vi "Initialize.vi"(8 "error in (no error)":errorcluster, 9 "id query (False)":bool caption="id query (True)", 10 "reset device (False)":bool caption="reset device (True)", 11 "Simulation in":refnum<class "Simulation.lvclass">) -> (0 "error out":errorcluster, 3 "Simulation out":refnum<class "Simulation.lvclass">)   [LabVIEW 2018, in "DigitizerPlugins.lvlib" / "Simulation.lvclass"]
uses:
  Simulation.lvclass
  Y:/Projects/PMUCal/Modules/Digitizer/DigitizerPlugins/DigitizerBaseClass/DigitizerBase.lvclass
  FGen/MemberClasses/PmuTestFunctions/PmuTestConfig.ctl
  FGen/MemberClasses/ArbitraryFunction/TypeDefs/ArbCfg.ctl
  FGen/MemberClasses/ArbitraryFunction/TypeDefs/Arbitrary.ctl
  Simulation.lvclass/Simulation.ctl
  DigitizerBaseClass/DigitizerBase.lvclass/DigitizerBase.ctl
  Accessors/Read Function.vi
  DigitizerBaseClass/Accessors/Read Acquisition.vi
  Accessors/Write Function.vi
  FGen/MemberClasses/FunctionBaseClass/FunctionBase.lvclass
  FGen/MemberClasses/ArbitraryFunction/ArbitraryFunction.lvclass
  FGen/MemberClasses/PmuTestFunctions/PmuTestFunctions.lvclass
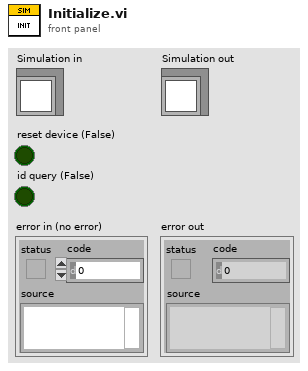
[diagram p1: front panel]
types:
  T1 = typedef "Functions.lvlib/PmuTestFunctions.lvclass/PmuTestConfig.ctl" = cluster{"T0":dbl, "SettlingTime":dbl, "ArbCfg":T2}
  T2 = typedef "Functions.lvlib/ArbitraryFunction.lvclass/ArbCfg.ctl" = cluster{"SampleRate":dbl, "Count":u16, "Arbs":T3[]}
  T3 = typedef "Functions.lvlib/ArbitraryFunction.lvclass/Arbitrary.ctl" = cluster{"Handle":string, "Size":i32, "Gain":dbl, "Offset":dbl, "Waveform":waveform(dbl)}
  T4 = typedef "DigitizerPlugins.lvlib/DigitizerBase.lvclass/Acquisition.ctl" = cluster{"SampleRate":dbl, "RecordSize":i32, "NumRecords":i32, "SampleMode":i32, "Timeout (ms)":i32}
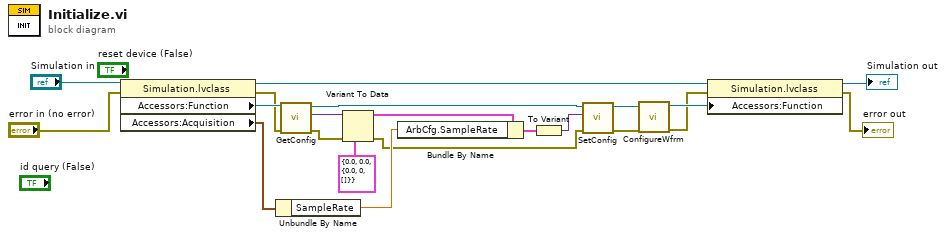
[diagram p0: block diagram]
diagram:
  n1 = property class="Simulation.lvclass"(reference="Simulation in", error in="error in (no error)") -> (reference out=w18:refnum<class "Simulation.lvclass">, error out=w12:errorcluster, "Accessors:Function"=w13:refnum<class "FunctionBase.lvclass">, "Accessors:Acquisition"=w14:T4)
  n2 = Unbundle By Name(w14) -> ("SampleRate"=w7:dbl)
  n3 = call-dynamic "GetConfig.vi"("error in (no error)"=w12, "FunctionBase in"=w13) -> ("error out"=w10:errorcluster, "Config"=w11:variant, "FunctionBase out"=w1:refnum<class "FunctionBase.lvclass">)  [unwired: 7 in]
  n4 = Variant To Data(error in=w10, type=T1 {"T0"=0.0, "SettlingTime"=0.0, "ArbCfg"={"SampleRate"=0.0, "Count"=0, "Arbs"=[]}} ("PmuTestConfig"), Variant=w11) -> (data=w8:T1, error out=w4:errorcluster)
  n5 = Bundle By Name(cluster=w8, "ArbCfg.SampleRate"=w7) -> (w6:T1)
  n6 = To Variant(anything=w6) -> (Variant=w5:variant)
  n7 = call-dynamic "SetConfig.vi"("error in (no error)"=w4, "Variant"=w5, "FunctionBase in"=w1) -> ("error out"=w3:errorcluster, "FunctionBase out"=w2:refnum<class "FunctionBase.lvclass">)  [unwired: 7 in]
  n8 = call-dynamic "ConfigureWfrm.vi"("error in (no error)"=w3, "FunctionBase in"=w2) -> ("error out"=w17:errorcluster, "FunctionBase out"=w19:refnum<class "FunctionBase.lvclass">)  [unwired: 8 in]
  n9 = property class="Simulation.lvclass"(reference=w18, error in=w17, "Accessors:Function"=w19) -> (reference out=→"Simulation out":refnum<class "Simulation.lvclass">, error out=→"error out":errorcluster)
